vi "NNF_Get_NN.vi"(11 "NNF in":T1) -> (3 "NN out":T7 {"LR_Update_Policy"."WarmUp_Ratio" min=1; "LR_Update_Policy"."WarmUp_Iter" min=1; "LR_Update_Policy"."LR0" format="%.7f"})   [LabVIEW 2020]
uses:
  <vilib>/Ngene/Deep Learning Toolkit/Toolkit/NN_Network/Controls/NN.ctl
  <vilib>/Ngene/Deep Learning Toolkit/Toolkit/NN_Layers/Controls/NN_Layer_ref.ctl
  <vilib>/Ngene/Deep Learning Toolkit/Toolkit/NN_Layers/Controls/NN_Layer.ctl
  <vilib>/Ngene/Deep Learning Toolkit/Toolkit/NN_Layers/Controls/NN_Layer_Type.ctl
  <vilib>/Ngene/Deep Learning Toolkit/Toolkit/NN_Data/API/NN_Dims(C,H,W).ctl
  <vilib>/Ngene/Deep Learning Toolkit/Toolkit/NN_Layers/Controls/NN_Layer_Metrics.ctl
  <vilib>/Ngene/Deep Learning Toolkit/Toolkit/NN_Network/Controls/NN_Device.ctl
  <vilib>/Ngene/Deep Learning Toolkit/Toolkit/NNg/cuda/Controls/nng_cuda_handles.ctl
  <vilib>/Ngene/Deep Learning Toolkit/Toolkit/NN_Layers/Controls/NN_Layer_Dimty.ctl
  <vilib>/Ngene/Deep Learning Toolkit/Toolkit/NN_Layers/Controls/NN_Layer_RF_State.ctl
  <vilib>/Ngene/Deep Learning Toolkit/Toolkit/NN_Data/API/NN_Dims(V,H).ctl
  <vilib>/Ngene/Deep Learning Toolkit/Toolkit/NN_Network/Controls/NN_In_Out_Dim-ty.ctl
  <vilib>/Ngene/Deep Learning Toolkit/Toolkit/NN_Train/Controls/NN_Train_Params.ctl
  <vilib>/Ngene/Deep Learning Toolkit/Toolkit/NN_Train/Controls/NN_Train_Optimizer.ctl
  <vilib>/Ngene/Deep Learning Toolkit/Toolkit/NN_Train/Controls/NN_Train_Data_Sampling.ctl
  <vilib>/Ngene/Deep Learning Toolkit/Toolkit/NN_Train/Controls/NN_LR_Policy_Cfg.ctl
  <vilib>/Ngene/Deep Learning Toolkit/Toolkit/NN_Train/Controls/NN_LR_Policy_Type.ctl
  <vilib>/Ngene/Deep Learning Toolkit/Toolkit/NN_Train/Controls/NN_Train_Session_Data.ctl
  <vilib>/Ngene/Deep Learning Toolkit/Toolkit/NN_Data/Controls/NN_Ground_truth.ctl
  <vilib>/Ngene/Deep Learning Toolkit/Toolkit/NN_Train/Controls/NN_Loss_Type.ctl
  <vilib>/Ngene/Deep Learning Toolkit/Toolkit/NNg/Network/WS/Controls/NNG_WS.ctl
  <vilib>/Ngene/Deep Learning Toolkit/Toolkit/NNg/Network/WS/Controls/NNg_WS_Mem_DVR.ctl
  <vilib>/Ngene/Deep Learning Toolkit/Toolkit/NNg/cuda/Controls/cuda_Mem_desc.ctl
  <vilib>/Ngene/DeepLTK FPGA Addon/Toolkit/NNF_Host/Low_Level/NNF_Common/Controls/NNF.ctl
  <vilib>/Ngene/DeepLTK FPGA Addon/Toolkit/NNF_Host/Low_Level/NNF_Common/Controls/NNF_Subnet.ctl
  <vilib>/Ngene/DeepLTK FPGA Addon/Toolkit/NNF_Host/Low_Level/NNF_Common/Controls/NNF_Subnet_Type.ctl
  <vilib>/Ngene/DeepLTK FPGA Addon/Toolkit/NNF_Host/Low_Level/NNF_Common/Controls/NNF_No_Of_Cores.ctl
  <vilib>/Ngene/DeepLTK FPGA Addon/Toolkit/NNF_Host/Low_Level/NNF_Common/Controls/NN_DVR.ctl
  <vilib>/Ngene/Deep Learning Toolkit/Toolkit/Deep_Learning_Toolkit_by_Ngene.lvlib
  <vilib>/Ngene/DeepLTK FPGA Addon/Toolkit/DeepLTK_FPGA_Addon.lvlib
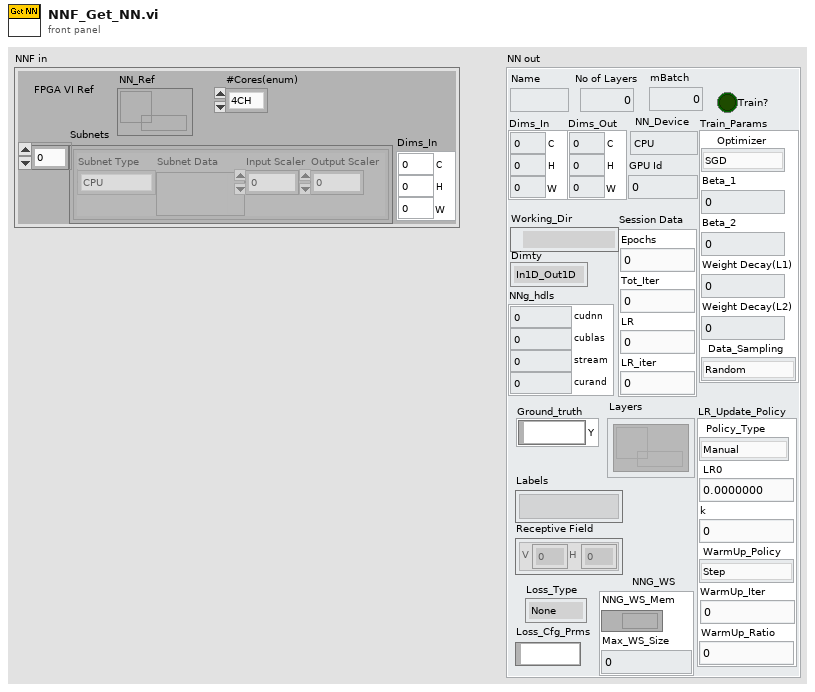
[diagram p1: front panel]
types:
  T1 = typedef "DeepLTK_FPGA_Addon.lvlib/NNF.ctl" = cluster{"FPGA VI Ref ":refnum<k20>, "Subnets":T2[], "Dims_In":T4, "#Cores(enum)":T5, "NN_Ref":T6}
  T2 = typedef "DeepLTK_FPGA_Addon.lvlib/NNF_Subnet.ctl" = cluster{"Subnet Type":T3, "Subnet Data":variant, "Input Scaler":sgl, "Output Scaler":sgl}
  T3 = typedef "DeepLTK_FPGA_Addon.lvlib/NNF_Subnet_Type.ctl" = enum16{"CPU", "FPGA", "Split FPGA"}
  T4 = typedef "Deep_Learning_Toolkit_by_Ngene.lvlib/NN_Dims(C,H,W).ctl" = cluster{"C":i32, "H":i32, "W":i32}
  T5 = typedef "DeepLTK_FPGA_Addon.lvlib/NNF_No_Of_Cores.ctl" = enum16{"4CH", "8CH"}
  T6 = typedef "DeepLTK_FPGA_Addon.lvlib/NN_DVR.ctl" = refnum<data-value>
  T7 = typedef "Deep_Learning_Toolkit_by_Ngene.lvlib/NN.ctl" = cluster{"Name":string, "No of Layers":i32, "mBatch":i32, "Layers":T8[], "Dimty":T9, "Dims_In":T4, "Dims_Out":T4, "Working_Dir":path, "Train?":bool, "Train_Params":T10, "LR_Update_Policy":T13, "Session Data":T15, "Ground_truth":T16, "NNg_hdls":T17, "NN_Device":T18, "GPU Id":i32, "Labels":string[], "Receptive Field":T19[], "Loss_Type":T20, "Loss_Cfg_Prms":variant, "NNG_WS":T21}
  T8 = typedef "Deep_Learning_Toolkit_by_Ngene.lvlib/NN_Layer_ref.ctl" = refnum<data-value>
  T9 = typedef "Deep_Learning_Toolkit_by_Ngene.lvlib/NN_In_Out_Dim-ty.ctl" = enum8{"In1D_Out1D", "In3D_Out1D", "In3D_Out3D", "In3D_OutBBox"}
  T10 = typedef "Deep_Learning_Toolkit_by_Ngene.lvlib/NN_Train_Params.ctl" = cluster{"Optimizer":T11, "Beta_1":sgl, "Beta_2":sgl, "Weight Decay(L1)":sgl, "Weight Decay(L2)":sgl, "Data_Sampling":T12}
  T11 = typedef "Deep_Learning_Toolkit_by_Ngene.lvlib/NN_Train_Optimizer.ctl" = enum16{"SGD", "Adam", "Adagrad", "Adadelta", "RMSProp", "Nesterov"}
  T12 = typedef "Deep_Learning_Toolkit_by_Ngene.lvlib/NN_Train_Data_Sampling.ctl" = enum16{"Random", "Sequential"}
  T13 = typedef "Deep_Learning_Toolkit_by_Ngene.lvlib/NN_LR_Policy_Cfg.ctl" = cluster{"Policy_Type":T14, "LR0":dbl, "k":sgl, "WarmUp_Policy":enum16{"Step", "Ramp"}, "WarmUp_Iter":i32, "WarmUp_Ratio":sgl}
  T14 = typedef "Deep_Learning_Toolkit_by_Ngene.lvlib/NN_LR_Policy_Type.ctl" = enum16{"Manual", "Step", "Exp", "1/t"}
  T15 = typedef "Deep_Learning_Toolkit_by_Ngene.lvlib/NN_Train_Session_Data.ctl" = cluster{"Epochs":sgl, "Tot_Iter":i32, "LR":sgl, "LR_iter":i32}
  T16 = typedef "Deep_Learning_Toolkit_by_Ngene.lvlib/NN_Ground_truth.ctl" = cluster{"Y":variant}
  T17 = typedef "Deep_Learning_Toolkit_by_Ngene.lvlib/nng_cuda_handles.ctl" = cluster{"cudnn":u64, "cublas":u64, "stream":u64, "curand":u64}
  T18 = typedef "Deep_Learning_Toolkit_by_Ngene.lvlib/NN_Device.ctl" = enum16{"CPU", "GPU"}
  T19 = typedef "Deep_Learning_Toolkit_by_Ngene.lvlib/NN_Dims(V,H).ctl" = cluster{"V":i32, "H":i32}
  T20 = typedef "Deep_Learning_Toolkit_by_Ngene.lvlib/NN_Loss_Type.ctl" = enum16{"None", "MSE", "CrossEntropy", "YOLO_v2", "YOLO_v4"}
  T21 = typedef "Deep_Learning_Toolkit_by_Ngene.lvlib/NNG_WS.ctl" = cluster{"NNG_WS_Mem":T22, "Max_WS_Size":i64}
  T22 = typedef "Deep_Learning_Toolkit_by_Ngene.lvlib/NNg_WS_Mem_DVR.ctl" = refnum<data-value>
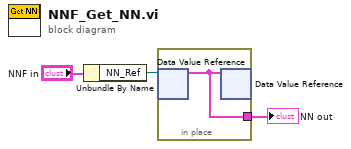
[diagram p0: block diagram]
diagram:
  n1 = Unbundle By Name("NNF in") -> ("NN_Ref"=w1:T6)
  n2 = in-place {
    in-place-border: [w4] -> w3
    n3 = in-place-dvr #1(w1) -> (w4:T7)  [unwired: 1 out]
    n4 = in-place-dvr #1(w4) -> ()  [unwired: 2 out]
  }
  "NN out" <- w3
